vi "read_DAW_ex.vi"() -> ()   [LabVIEW 2019]
panel:
  out "Numeric 4":dbl
  out "Numeric 3":dbl
  out "Numeric 2":dbl
  out "Numeric":dbl
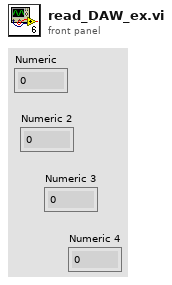
[diagram p1: front panel]
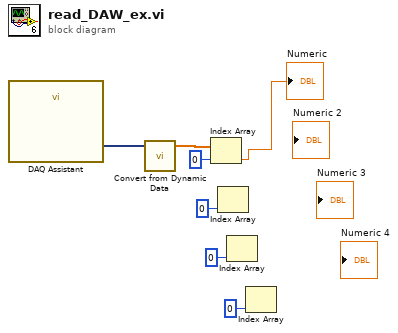
[diagram p0: block diagram]
diagram:
  n1 = call "DAQ Assistant"() -> ("data"=w7:dynamicdata)  [unwired: 17 in, 2 out]
  n2 = call "Convert from Dynamic Data"("Dynamic Data Type"=w7) -> ("Array"=w6:dbl[])  [unwired: 3 in]
  n3 = Index Array(array=w6, index=0) -> (element=→"Numeric":dbl)
  n4 = Index Array(index=0) -> ()  [unwired: 1 in, 1 out]
  n5 = Index Array(index=0) -> ()  [unwired: 1 in, 1 out]
  n6 = Index Array(index=0) -> ()  [unwired: 1 in, 1 out]
